vi "Check ACQ Status (test).vi"(0 "device session in":refnum<class "Device Session.lvclass">, 1 "Fetch?":bool, 5 "record number":u64, 7 "fetch relative to":T4, 9 "fetch offset":i64, 11 "error in":errorcluster) -> (2 "done":bool, 3 "record status":T2, 4 "device session out":refnum<class "Device Session.lvclass">, 6 "fetch backlog":u64, 8 "number of outstanding record requests":u32, 10 "records done":u64, 13 "overflow occurred":bool, 14 "current record status":T1, 15 "error out":errorcluster)   [LabVIEW 2021, in "Device Session.lvclass"]
doc: "Checks the overall status of the device and reports whether it is operating correctly. This VI checks for system monitor alarms, such as temperature error, power error, FPGA voltage errors, clock PLL lock errors, and channel overload errors.\n\n<B>Input Parameters</B>\n\n<B>device session in</B> is a reference to the Device Session object, which contains a session to each instrument design library used in this sample project. This parameter is obtained from the 'Open Session' VI.\n\n<B>error in</B> describes error conditions that occur before this node runs. This input provides standard 'error in' functionality.\n\n<B>Output Parameters</B>\n\n<B>device session out</B> passes a reference to the session to the next VI.\n\n<B>error out</B> contains error information. This output provides standard 'error out' functionality."
uses:
  Device Session.lvclass
  <instrlib>/_niInstr/Multirecord Acquisition/Interface/v1/Host/Public/Fetch Relative To Enum.ctl
  <instrlib>/_niInstr/Multirecord Acquisition/Interface/v1/Host/Public/Full Record Status.ctl
  <instrlib>/_niInstr/Multirecord Acquisition/Interface/v1/Host/Public/Record State.ctl
  <instrlib>/_niInstr/Multirecord Acquisition/Interface/v1/Host/Public/Record Status.ctl
  Device Session.lvclass/Device Session.ctl
  <instrlib>/_niInstr/Multirecord Acquisition/Interface/v1/Host/niInstr Multirecord Acquisition v1 Host.lvclass
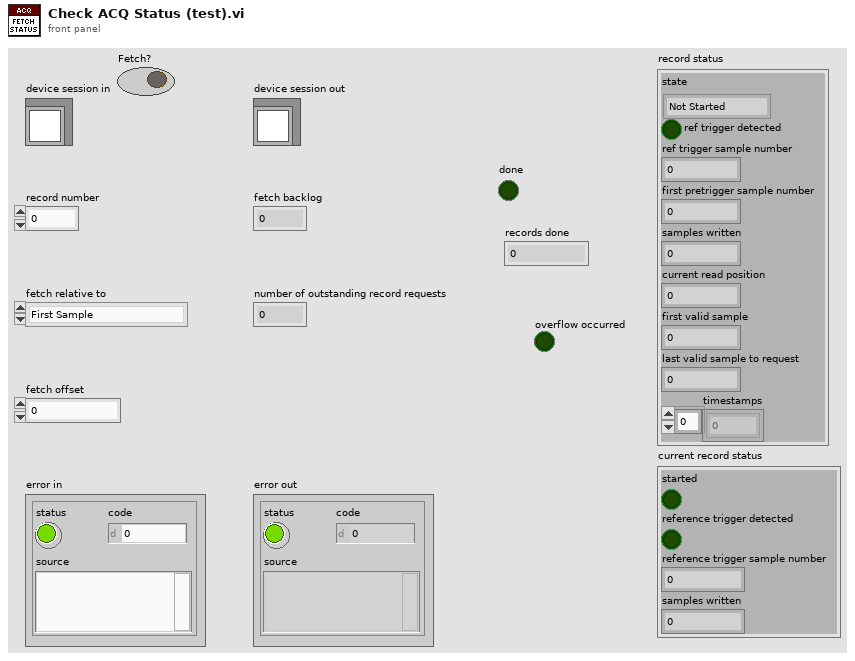
[diagram p1: front panel]
types:
  T1 = typedef "niInstr Multirecord Acquisition v1 Host.lvclass/Record Status.ctl" = cluster{"started":bool, "reference trigger detected":bool, "reference trigger sample number":u64, "samples written":u64}
  T2 = typedef "niInstr Multirecord Acquisition v1 Host.lvclass/Full Record Status.ctl" = cluster{"state":T3, "ref trigger detected":bool, "ref trigger sample number":u64, "first pretrigger sample number":u64, "samples written":u64, "current read position":u64, "first valid sample":u64, "last valid sample to request":u64, "timestamps":u64[]}
  T3 = typedef "niInstr Multirecord Acquisition v1 Host.lvclass/Record State.ctl" = enum16{"Not Started", "Being Acquired", "Completed", "Overwritten"}
  T4 = typedef "niInstr Multirecord Acquisition v1 Host.lvclass/Fetch Relative To Enum.ctl" = enum16{"First Sample", "Reference Trigger Sample", "First Pretrigger Sample", "Most Recent Sample", "Current Read Position"}
  T5 = typedef "Device Session.lvclass/Device Session Object.ctl" = cluster{"fpga reference":T6, "reg bus":refnum<class "niInstr FIFO Register Bus v1 Host.lvclass">, "subsystem map":refnum<class "niInstr Subsystem Map v1 Host.lvclass">, "cal data":refnum<class "niHSAI Cal Data v1 Host.lvclass">, "config":refnum<class "niHSAI Group A Config v1 Host.lvclass">, "acquisition":refnum<class "niInstr Multirecord Acquisition v1 Host.lvclass">, "number of selected acq channels":u8, "selected acq channels":bool[], "number of channels":u32, "configured channels":bool[], "acq configuration":cluster{"number of samples":u64, "number of records":u64, "pretrigger samples":u64}, "actual channel configuration":T7[], "sample clock rate (Hz)":dbl, "scaling coefficients":T11[]}
  T6 = typedef "Device Session.lvclass/FPGA Refnum.ctl" = refnum<k20>
  T7 = typedef "niHSAI Types v1 Host.lvlib/Channel Configuration.ctl" = cluster{"channel":u32, "coupling":T8, "impedance":T9, "bandwidth":T10, "vertical range":dbl, "vertical offset":dbl}
  T8 = typedef "niHSAI Types v1 Host.lvlib/Coupling.ctl" = enum8{"Default", "DC", "AC"}
  T9 = typedef "niHSAI Types v1 Host.lvlib/Impedance.ctl" = enum8{"Default", "1 mega ohm", "50 ohm"}
  T10 = typedef "niHSAI Types v1 Host.lvlib/Bandwidth.ctl" = enum8{"Default", "Full Bandwidth", "Anti-alias Filter", "150 MHz"}
  T11 = typedef "niInstr Multirecord Acquisition v1 Host.lvclass/Scaling Coefficient.ctl" = cluster{"gain":dbl, "offset":dbl}
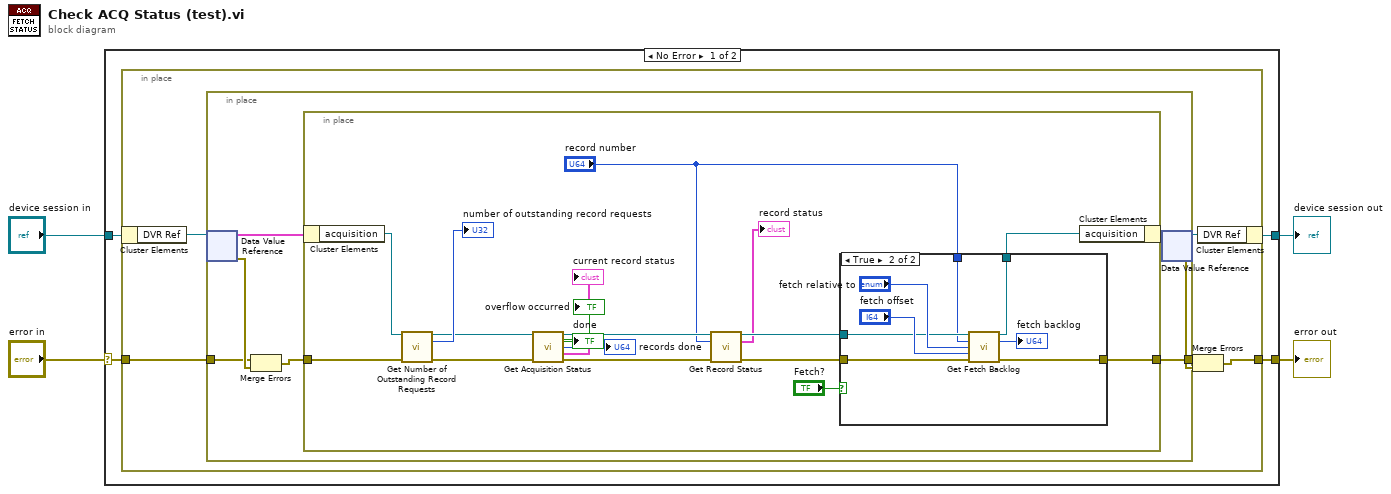
[diagram p0: block diagram]
diagram:
  n1 = case shown="No Error" "error in" {
    selector: "error in" -> [w8 w50]
    tunnel: "device session in" -> [w6 w49]
    tunnel: [w5 w49] -> w2
    tunnel: [w7 w50] -> w1
    frame No Error {
      n2 = in-place {
        in-place-border: w8 -> [w14]
        in-place-border: [w11] -> w7
        n3 = in-place-cluster #1(w6) -> ("DVR Ref"=w10:refnum<data-value>)
        n4 = in-place {
          in-place-border: w14 -> [w17]
          in-place-border: [w20] -> w12
          n5 = in-place-dvr #2(w10) -> (w16:T5, w18:errorcluster)
          n6 = Merge Errors(w17, w18) -> (w19:errorcluster)
          n7 = in-place {
            in-place-border: [w38] -> w20
            in-place-border: w19 -> [w35]
            n8 = in-place-cluster #3(w16) -> ("acquisition"=w36:refnum<class "niInstr Multirecord Acquisition v1 Host.lvclass">)
            n9 = call-dynamic "Get Number of Outstanding Record Requests.vi"("session in"=w36, "error in"=w35) -> ("session out"=w29:refnum<class "niInstr Multirecord Acquisition v1 Host.lvclass">, "number of outstanding record requests"=→"number of outstanding record requests":u32, "error out"=w28:errorcluster)  [unwired: 11 in]
            n10 = call-dynamic "Get Acquisition Status.vi"("session in"=w29, "error in"=w28) -> ("overflow occurred"=→"overflow occurred":bool, "session out"=w33:refnum<class "niInstr Multirecord Acquisition v1 Host.lvclass">, "done"=→"done":bool, "records done"=→"records done":u64, "current record status"=→"current record status":T1, "error out"=w32:errorcluster)  [unwired: 8 in]
            n11 = call-dynamic "Get Record Status.vi"("session in"=w33, "record number"="record number", "error in"=w32) -> ("session out"=w31:refnum<class "niInstr Multirecord Acquisition v1 Host.lvclass">, "record status"=→"record status":T2, "error out"=w30:errorcluster)  [unwired: 10 in]
            n12 = case shown="True" "Fetch?" {
              tunnel: [w39 w48] -> w38
              tunnel: [w40 w47] -> w37
              tunnel: w31 -> [w40 w43]
              tunnel: w30 -> [w39 w42]
              tunnel: "record number" -> [_ w41]
              frame False {
              }
              frame True {
                n13 = call-dynamic "Get Fetch Backlog.vi"("session in"=w43, "record number"=w41, "fetch relative to"="fetch relative to", "fetch offset"="fetch offset", "error in"=w42) -> ("session out"=w47:refnum<class "niInstr Multirecord Acquisition v1 Host.lvclass">, "fetch backlog"=→"fetch backlog":u64, "error out"=w48:errorcluster)  [unwired: 8 in]
              }
            }
            n14 = in-place-cluster #3("acquisition"=w37) -> (w15:T5)
          }
          n15 = in-place-dvr #2(w15) -> (w9:refnum<data-value>, w13:errorcluster)
        }
        n16 = Merge Errors(w12, w13) -> (w11:errorcluster)
        n17 = in-place-cluster #1("DVR Ref"=w9) -> (w5:refnum<class "Device Session.lvclass">)
      }
    }
    frame Error {
    }
  }
  "error out" <- w1
  "device session out" <- w2
